vi "TEST_ASIC_MAJnADDS_NEWII.vi"(5 "threshold":i32[][](array[numeric])=[[520, 516, 524, 514, 514, 514, 524], [524, 526, 526, 516, 518, 516, 528], [534, 530, 532, 518, 526, 532, 532], [540, 538, 532, 534, 536, 532, 544], [534, 550, 550, 544, 546, 528, 538]], 7 "Serial Number":string="SN_903", 8 "error in":errorcluster, 11 "Instrument VISA in":T1={"AWG VISA"="AgilentGenerator1", "Oscilloscope  VISA "="AgilentOsciloscope", "Integration Board IP"="172.16.17.47", "connection ID"=refnum, "report out"=refnum, "report file path"=path "C:/Users/omartinez/Desktop/L0nL1_Results"}) -> (0 "error out":errorcluster, 3 "Instrument VISA out":T1={"AWG VISA"="AgilentGenerator1", "Oscilloscope  VISA "="AgilentOsciloscope", "Integration Board IP"="172.16.17.47", "connection ID"=refnum, "report out"=refnum, "report file path"=path "C:/Users/omartinez/Desktop/L0nL1_Results"})   [LabVIEW 2012]
uses:
  <vilib>/Utility/NIReport.llb/NI_report.lvclass
  <vilib>/Utility/NIReport.llb/HTML/NI_HTML.lvclass
  <instrlib>/Agilent 8000 Series/Public/Configure/Configure Math (Binary Operation).vi
  Sum_Abrilader/L0_Sum_Adder Folder/C/Program Files/National Instruments/LabVIEW 2012/instr.lib/Agilent 8000 Series/Public/Data/Low Level/Fetch Measurement (More).vi
  Sum_Abrilader/L0_Sum_Adder Folder/C/Program Files/National Instruments/LabVIEW 2012/instr.lib/Agilent 81150/Agilent 81150.lvlib
  <instrlib>/Agilent 8000 Series/Agilent 8000 Series.lvlib
panel:
  in  "Channels \nCombinations":i32[](array[numeric])=[3, 12, 48, 96, 7, 28, 112, 15, 120, 31, 124, 63, 126, 127]
  in  "Voltages":dbl[](array[numeric])=[0.05, 0.1, 0.2, 0.5, 0.8]
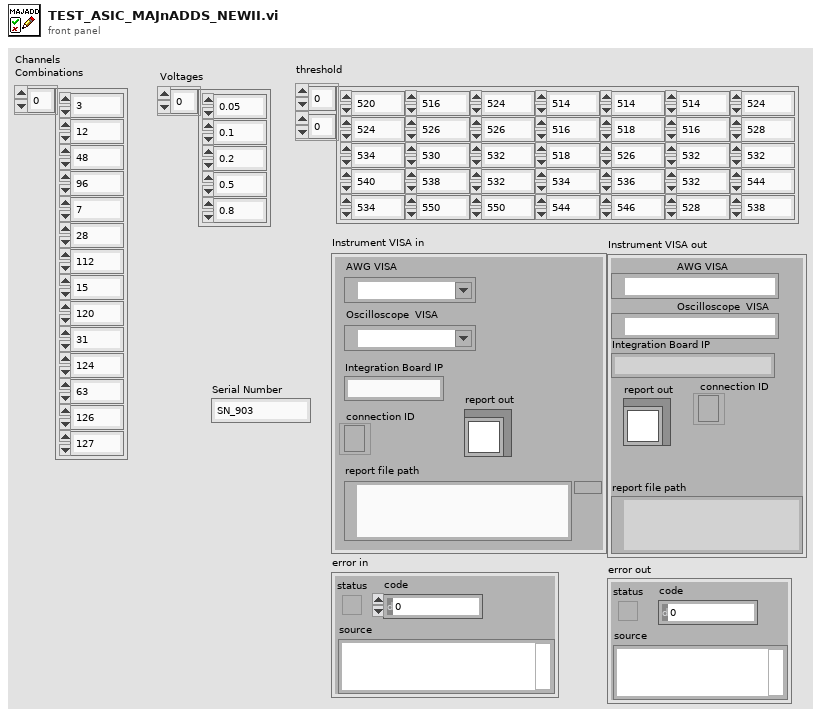
[diagram p1: front panel]
types:
  T1 = cluster{"AWG VISA":refnum<visa-resource-name>, "Oscilloscope  VISA ":refnum<visa-resource-name>, "Integration Board IP":string, "connection ID":refnum<k5>, "report out":refnum<class "NI_report.lvclass">, "report file path":path}
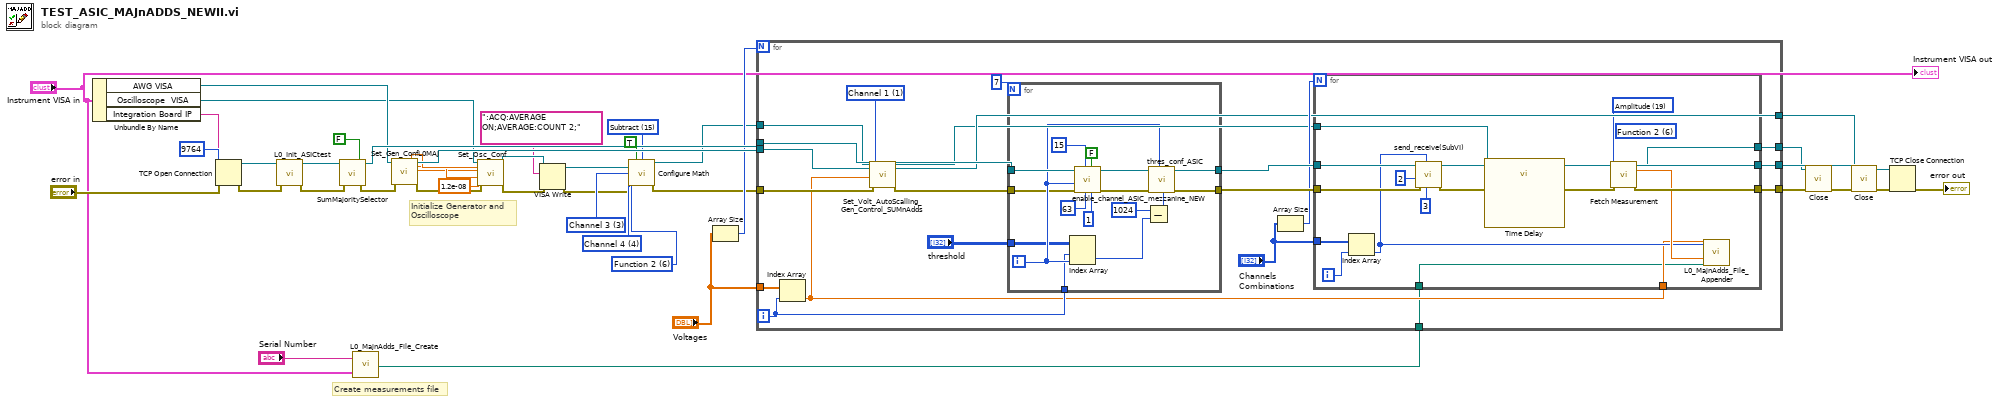
[diagram p0: block diagram]
diagram:
  w22 = u16 6 items=["Function 1"=5, "Function 2"=6, "Function 3"=7, "Function 4"=8] ("Math Channel (5: Function 1)")
  w23 = u16 15 items=["Add"=12, "Divide"=13, "Multiply"=14, "Subtract"=15, "Common Mode"=16, "Versus"=17] ("Math Operation (12: Add)")
  w21 = 3 items=["Channel 1"=1, "Channel 2"=2, "Channel 3"=3, "Channel 4"=4] ("Channel (1: Channel 1)")
  w20 = 4 items=["Channel 1"=1, "Channel 2"=2, "Channel 3"=3, "Channel 4"=4] ("Channel (1: Channel 1)")
  # "Create measurements file"
  # "Initialize Generator and \nOscilloscope"
  n1 = Unbundle By Name("Instrument VISA in") -> ("AWG VISA"=w30:refnum<visa-resource-name>, "Oscilloscope  VISA"=w14:refnum<visa-resource-name>, "Integration Board IP"=w41:string)
  n2 = TCP Open Connection(address=w41, remote port or service name=9764, error in (no error)="error in") -> (connection ID=w36:refnum<k5>, error out=w37:errorcluster)  [unwired: 2 in]
  n3 = call "L0_Init_ASICtest.vi"("error in"=w37, "connection ID in"=w36) -> ("error out"=w38:errorcluster, "connection ID out"=w35:refnum<k5>)  [unwired: 8 in]
  n4 = call "SumMajoritySelector.vi"("On Sum\nOff Majority"=FALSE ("On Sum\nOff Majority"), "error in (no error)"=w38, "connection ID"=w35) -> ("error out"=w32:errorcluster, "connection ID out"=w31:refnum<k5>)  [unwired: 5 in]
  n5 = call "L0_MajnAdds_File_Create.vi"("input cluster"="Instrument VISA in", "Serial Number"="Serial Number") -> ("appended path"=w5:path)
  n6 = call "Set_Gen_ConfL0MAJ.vi"("AWG VISA"=w30, "error in (no error)"=w32) -> ("Amplitude 1 OUT"=w11:dbl, "VISA resource name out"=w29:refnum<visa-resource-name>, "Pulse Width in seconds 1 OUT"=w10:dbl, "Trigger Level 1"=w9:dbl, "error out"=w13:errorcluster)  [unwired: 10 in, 3 out]
  n7 = call "Set_Osc_Conf.vi"("VISA resource name"=w14, "Amplitude IN"=w11, "Trigger Level IN"=w9, "Pulse Width in seconds IN"=w10, "Position 1"=1.2e-08, "error in (no error)"=w13) -> ("VISA resource name out"=w18:refnum<visa-resource-name>, "error out"=w19:errorcluster)  [unwired: 12 in]
  n8 = VISA Write(VISA resource name=w18, write buffer=":ACQ:AVERAGE ON;AVERAGE:COUNT 2;", error in (no error)=w19) -> (VISA resource name out=w17:refnum<visa-resource-name>, error out=w16:errorcluster)  [unwired: 1 out]
  n9 = call-poly <instrlib>:"Configure Math.vi"("VISA resource name"=w17, "Enable Math Channel (T:Enable)"=TRUE, "Math Operation (12: Add)"=w23, "Math Channel (5: Function 1)"=w22, "Math Operand (1: Channel 1)"=w21, "Math Operand (2: Channel 2)"=w20, "error in (no error)"=w16) -> ("VISA resource name out"=w8:refnum<visa-resource-name>, "error out"=w12:errorcluster)  [unwired: 7 in]
  n10 = Array Size(array="Voltages") -> (size(s)=w25:i32)
  n11 = for {
    N: w25 -> [_]
    tunnel: [w63] -> w33
    tunnel: w31 -> [w62]
    tunnel: w12 -> [w49]
    tunnel: "Voltages" -> [w61]
    tunnel: w29 -> [w51]
    tunnel: [w60] -> w4
    tunnel: [w47] -> w27
    tunnel: w8 -> [w50]
    tunnel: w5 -> [w45]
    tunnel: [w43] -> w2
    i -> [w55]
    w52 = 1 items=["Channel 1"=1, "Channel 2"=2, "Channel 3"=3, "Channel 4"=4] ("Channel")
    n12 = Index Array(array=w61, index=w55) -> (element=w46:dbl)
    n13 = call "Set_Volt_AutoScalling_Gen_Control_SUMnAdds.vi"("VISA Oscilloscope"=w50, "VISA Generator"=w51, "Channel"=w52, "Amplitude"=w46, "error in (no error)"=w49) -> ("VISA Oscilloscope"=w44:refnum<visa-resource-name>, "VISA Generator"=w47:refnum<visa-resource-name>, "error out"=w48:errorcluster)  [unwired: 12 in]
    n14 = for {
      N: 7 -> [_]
      tunnel: [w97] -> w57
      tunnel: w62 -> [w95]
      tunnel: [w93] -> w56
      tunnel: "threshold" -> [w87]
      tunnel: w55 -> [w85]
      tunnel: w48 -> [w84]
      i -> [w88]
      n15 = Index Array(array=w87, index (row)=w85, index (col)=w88) -> (element=w86:i32)
      n16 = call "enable_channel_ASIC_mezzanine_NEW.vi"("Clip_sel_b"=u32 1, "maj/sum"=FALSE, "Ib_clipVb"=u32 63, "Att gain"=u32 15, "error in"=w84, "Channel"=w88, "connection ID"=w95) -> ("error out"=w96:errorcluster, "connection ID out"=w94:refnum<k5>)  [unwired: 2 in, 1 out]
      n17 = Subtract(x=1024, y=w86) -> (x-y=w83:i32)
      n18 = call "thres_conf_ASIC.vi"("threshold"=w83, "Ring"=w88, "error out 3"=w96, "connection ID"=w94) -> ("error out 2"=w97:errorcluster, "connection ID out"=w93:refnum<k5>)  [unwired: 4 in, 2 out]
    }
    n19 = Array Size(array="Channels \nCombinations") -> (size(s)=w53:i32)
    n20 = for {
      N: w53 -> [_]
      tunnel: [w81] -> w63
      tunnel: [w74] -> w60
      tunnel: w57 -> [w80]
      tunnel: w56 -> [w79]
      tunnel: "Channels \nCombinations" -> [w75]
      tunnel: w44 -> [w73]
      tunnel: w46 -> [w69]
      tunnel: w45 -> [w68]
      tunnel: [w64] -> w43
      i -> [w76]
      w67 = 6 items=["Channel 1"=1, "Channel 2"=2, "Channel 3"=3, "Channel 4"=4, "Function 1"=5, "Function 2"=6, "Function 3"=7, "Function 4"=8, "Memory 1"=9, "Memory 2"=10, "Memory 3"=11, "Memory 4"=12] ("Channel (1: Channel 1)")
      w72 = 19 items=["Rise Time", "Fall Time", "Frequency", "Period", "Voltage RMS(AC)", "Voltage RMS(DC)", "Voltage RMS (AC,cycle)", "Voltage RMS (DC,cycle)", "Voltage Max", "Voltage Min", "Voltage Middle", "Voltage Vpp", "Voltage High", "Voltage Low", "Voltage Average", "Voltage Average (cycle)", "Width Negative", "Width Positive", "Duty Cycle Positive", "Amplitude", "Overshoot", "Preshoot", "Voltage Base", "Voltage Upper", "Time Max", "Time Min", "Color Grade Crossing", "Color Grade Eye Width", "Color Grade Eye Height", "Color Grade Eye Q-Factory", "Color Grade Eye Duty Cycle Distortion(Percent)", "Color Grade Eye Duty Cycle Distortion(Time)", "Color Grade Eye Jitter(PP)", "Color Grade Eye Width(RMS)", "Cycle-cycle Duty Jitter(Rising)", "Cycle-cycle Duty Jitter(Falling)", "Cycle-cycle Jitter(Rising)", "Cycle-cycle Jitter(Falling)", "Cycle-cycle - Width", "Cycle-cycle + Width", "Date Rate", "Unit Interval", "FFT Delta Frequency", "FFT Delta Magnitude", "FFT Frequency", "FFT Magnitude", "Slew Rate", "Area (Entire Display)", "Area(Single Cycle)", "Duty Cycle (Rising)", "Duty Cycle (Falling)"] ("Measurement Function (0: Rise Time)")
      n21 = Index Array(array=w75, index=w76) -> (element=w70:i32)
      n22 = call "send_receive(SubVI).vi"("Action"=3, "Data"=w70, "error in"=w80, "Address"=2, "connection ID"=w79) -> ("error out"=w66:errorcluster, "connection ID out"=w81:refnum<k5>)  [unwired: 2 in, 3 out]
      n23 = call "Time Delay"("error in (no error)"=w66) -> ("error out"=w65:errorcluster)  [unwired: 10 in]
      n24 = call-poly "Fetch Measurement.vi"("VISA resource name"=w73, "Channel (1: Channel 1)"=w67, "Measurement Function (0: Rise Time)"=w72, "error in (no error)"=w65) -> ("VISA resource name out"=w64:refnum<visa-resource-name>, "Measurement"=w71:dbl, "error out"=w74:errorcluster)  [unwired: 9 in]
      n25 = call "L0_MajnAdds_File_Appender.vi"("Vin"=w69, "CH"=w70, "Vmeas"=w71, "file path (dialog if empty)"=w68) -> ()  [unwired: 24 in]
    }
  }
  n26 = call <instrlib>:"Close.vi"("error in (no error)"=w4, "VISA resource name"=w2) -> ("error out"=w3:errorcluster)  [unwired: 9 in]
  n27 = call <instrlib>:"Close.vi"("error in (no error)"=w3, "VISA resource name"=w27) -> ("error out"=w28:errorcluster)  [unwired: 9 in]
  n28 = TCP Close Connection(connection ID=w33, error in (no error)=w28) -> (error out=→"error out":errorcluster)  [unwired: 1 in, 1 out]
  "Instrument VISA out" <- "Instrument VISA in"
